vi "Get Actor VI Name.vi"() -> (0 "Actor VI Name":string)   [LabVIEW 2020, in "Msg.lvlib"]
doc: "Get the Actor Core Clone VI name using the call chain."
uses:
  Msg.lvlib
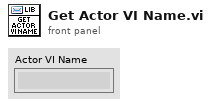
[diagram p1: front panel]
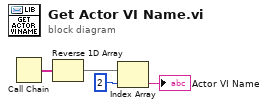
[diagram p0: block diagram]
diagram:
  n1 = Call Chain() -> (call chain=w4:string[])
  n2 = Reverse 1D Array(array=w4) -> (reversed array=w3:string[])
  n3 = Index Array(array=w3, index=2) -> (element=→"Actor VI Name":string)
